vi "Populate Cluster.vi"(5 "Force Data Conversion? (F)":bool, 7 "prefix":string, 8 "error in (no error)":errorcluster, 10 "data in":variant, 11 "Map":map{string, variant}(c390)) -> (0 "error out":errorcluster, 2 "data out":variant, 4 "all found?":bool, 6 "found tags":string[](array[string]))   [LabVIEW 2021, in "uData.lvlib" / "uData.lvclass"]
doc: "This is a recursive subVI to populate cluster elements."
uses:
  uData.lvclass
  <vilib>/Utility/error.llb/Error Cluster From Error Code.vi
  <vilib>/ErrorRing/Error Ring.xnode
  uData.lvclass/uData.ctl
  <vilib>/Utility/Data Type/NI_Data Type.lvlib
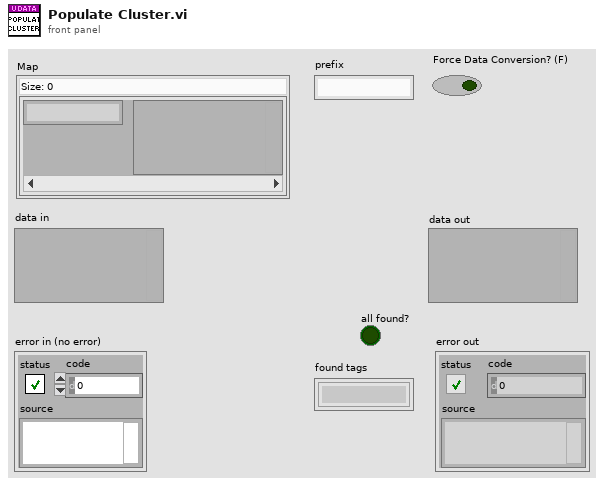
[diagram p1: front panel]
types:
  T1 = typedef "NI_Data Type.lvlib/Data Type.ctl" = enum8{"Invalid Type", "Void", "I8", "I16", "I32", "I64", "U8", "U16", "U32", "U64", "Single Float", "Double Float", "Extended Float", "Single Complex", "Double Complex", "Extended Complex", "Enum U8", "Enum U16", "Enum U32", "Enum U64", "Single Float With Unit", "Double Float With Unit", "Extended Float With Unit", "Single Complex with Unit", "Double Complex with Unit", "Extended Complex with Unit", "Boolean", "String", "Path", "Picture", "Tag", "Array", "Cluster", "Variant", "LV Variant", "Waveform", "Timestamp", "Digital Waveform", "Digital Data", "ExpressData", "Refnum", "External Data", "VI", "Poly VI", "LabVIEW Class Instance", "Fixed Point", "Set Collection", "Map Collection"}
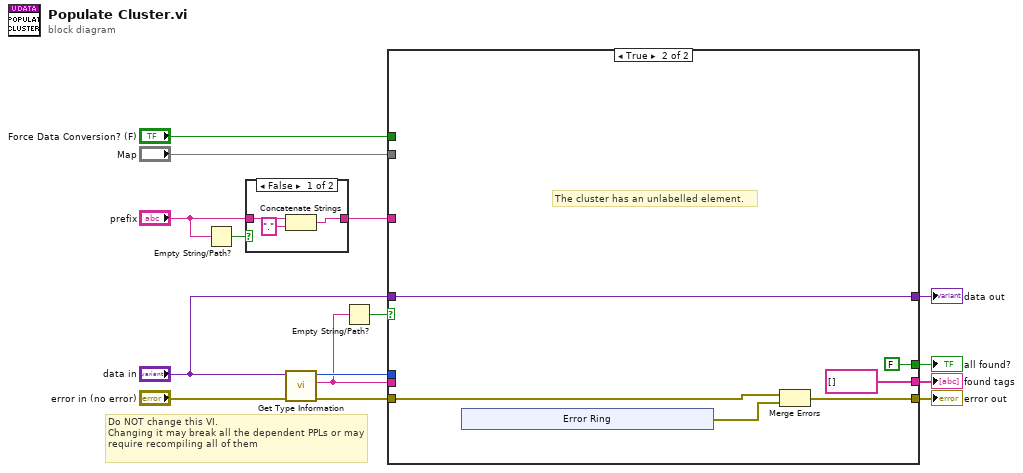
[diagram p0: block diagram]
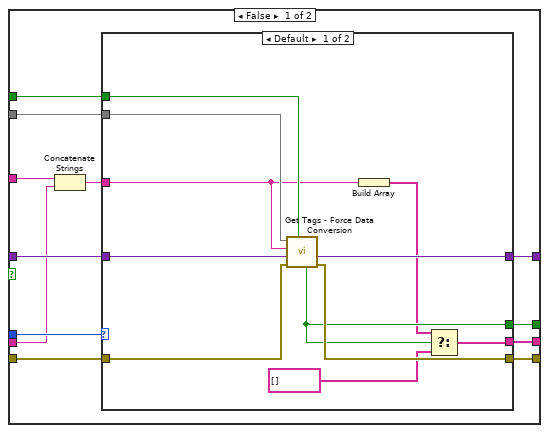
[diagram p3: hidden frame]
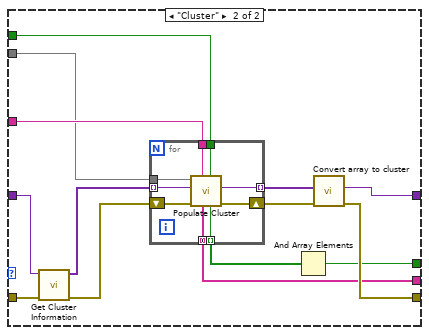
[diagram p4: hidden frame]
diagram:
  # "Do NOT change this VI.\nChanging it may break all the dependent PPLs or may require recompiling all of them"
  n1 = Empty String/Path?(string/path="prefix") -> (empty?=w6:bool)
  n2 = case shown="False" w6 {
    tunnel: "prefix" -> [w18 w19]
    tunnel: [w16 w19] -> w8
    frame False {
      n3 = Concatenate Strings(w18, "." ("string")) -> (w16:string)
    }
    frame True {
    }
  }
  n4 = call <vilib>:"Get Type Information.vi"("error in (no error)"="error in (no error)", "variant"="data in") -> ("error out"=w10:errorcluster, "name"=w7:string, "type"=w12:T1)  [unwired: 5 in, 2 out]
  n5 = Empty String/Path?(string/path=w7) -> (empty?=w3:bool)
  n6 = case shown="True" w3 {
    tunnel: "data in" -> [w31 w68]
    tunnel: w12 -> [w30 _]
    tunnel: [w29 w70] -> w11
    tunnel: w10 -> [w28 w71]
    tunnel: [w27 w68] -> w9
    tunnel: w7 -> [w26 _]
    tunnel: w8 -> [w25 _]
    tunnel: [w23 string[] [] ("found tags")] -> w5
    tunnel: [w22 FALSE ("all found?")] -> w4
    tunnel: "Force Data Conversion? (F)" -> [w21 _]
    tunnel: "Map" -> [w20 _]
    frame False {
      n7 = Concatenate Strings(w25, w26) -> (w24:string)
      n8 = case shown="Default" w30 {
        tunnel: w24 -> [w33 w56]
        tunnel: w28 -> [w42 w53]
        tunnel: w31 -> [w32 w55]
        tunnel: [w41 w50] -> w29
        tunnel: [w40 w49] -> w27
        tunnel: [w37 w47] -> w23
        tunnel: [w39 w45] -> w22
        tunnel: w21 -> [w35 w44]
        tunnel: w20 -> [w34 w43]
        frame Default {
          n9 = call "Get Tags - Force Data Conversion.vi"("Force Data Conversion? (F)"=w35, "error in (no error)"=w42, "default value"=w32, "key"=w33, "Map"=w34) -> ("error out"=w41:errorcluster, "value"=w40:variant, "found?"=w39:bool)  [unwired: 4 in]
          n10 = Build Array(w33) -> (w38:string[])
          n11 = Select(t=w38, s=w39, f=string[] []) -> (s? t:f=w37:string[])
        }
        frame "Cluster" {
          n12 = call <vilib>:"Get Cluster Information.vi"("error in (no error)"=w53, "variant"=w55) -> ("error out"=w54:errorcluster, "cluster elements"=w52:variant[])  [unwired: 8 in]
          n13 = for {
            tunnel: w43 -> [w65]
            tunnel: w56 -> [w64]
            shift-right: [w63] -> w51
            shift-left: w54 -> [w62]
            tunnel: w52 -> [w61] mode=indexing
            tunnel: [w60] -> w48 mode=indexing
            tunnel: [w59] -> w47 mode=concatenating
            tunnel: [w58] -> w46 mode=indexing
            tunnel: w44 -> [w57]
            n14 = call "Populate Cluster.vi"("Force Data Conversion? (F)"=w57, "prefix"=w64, "error in (no error)"=w62, "data in"=w61, "Map"=w65) -> ("error out"=w63:errorcluster, "data out"=w60:variant, "all found?"=w58:bool, "found tags"=w59:string[])  [unwired: 3 in]
          }
          n15 = And Array Elements(Boolean array=w46) -> (logical AND=w45:bool)
          n16 = call "Convert array to cluster.vi"("error in (no error)"=w51, "array"=w48) -> ("error out"=w50:errorcluster, "cluster"=w49:variant)  [unwired: 8 in]
        }
      }
    }
    frame True {
      # "The cluster has an unlabelled element."
      n17 = xnode "Error Ring"() -> ("error out"=w69:errorcluster)
      n18 = Merge Errors(w71, w69) -> (w70:errorcluster)
    }
  }
  "error out" <- w11
  "data out" <- w9
  "all found?" <- w4
  "found tags" <- w5
